vi "PathSup2ScanXML.vi"(3 "Thickness":dbl, 4 "Path":path, 5 "PathSupremes":T7[](array[typedef])) -> (2 "SCAN":T4)   [LabVIEW 2014]
uses:
  TypeDefs/PathSupreme.ctl
  Sub/VelocityProfile.ctl
  Sub/PathCut.ctl
  Sub/Segment.ctl
  TypeDefs/SCAN_XML.ctl
  Sub/Trajectory.ctl
  Sub/Path.ctl
  Sub/Point.ctl
  <vilib>/Utility/xml.llb/Write to XML File(string).vi
panel:
  out "xml string":string
  out "Path Supreames 2  String":string
  out "Trajectories Out":cluster{"TravelerID":u32, "SyncDelay":u32, T1[]}
  in  "SyncDelay":u32
  in  "TravelerID":u32
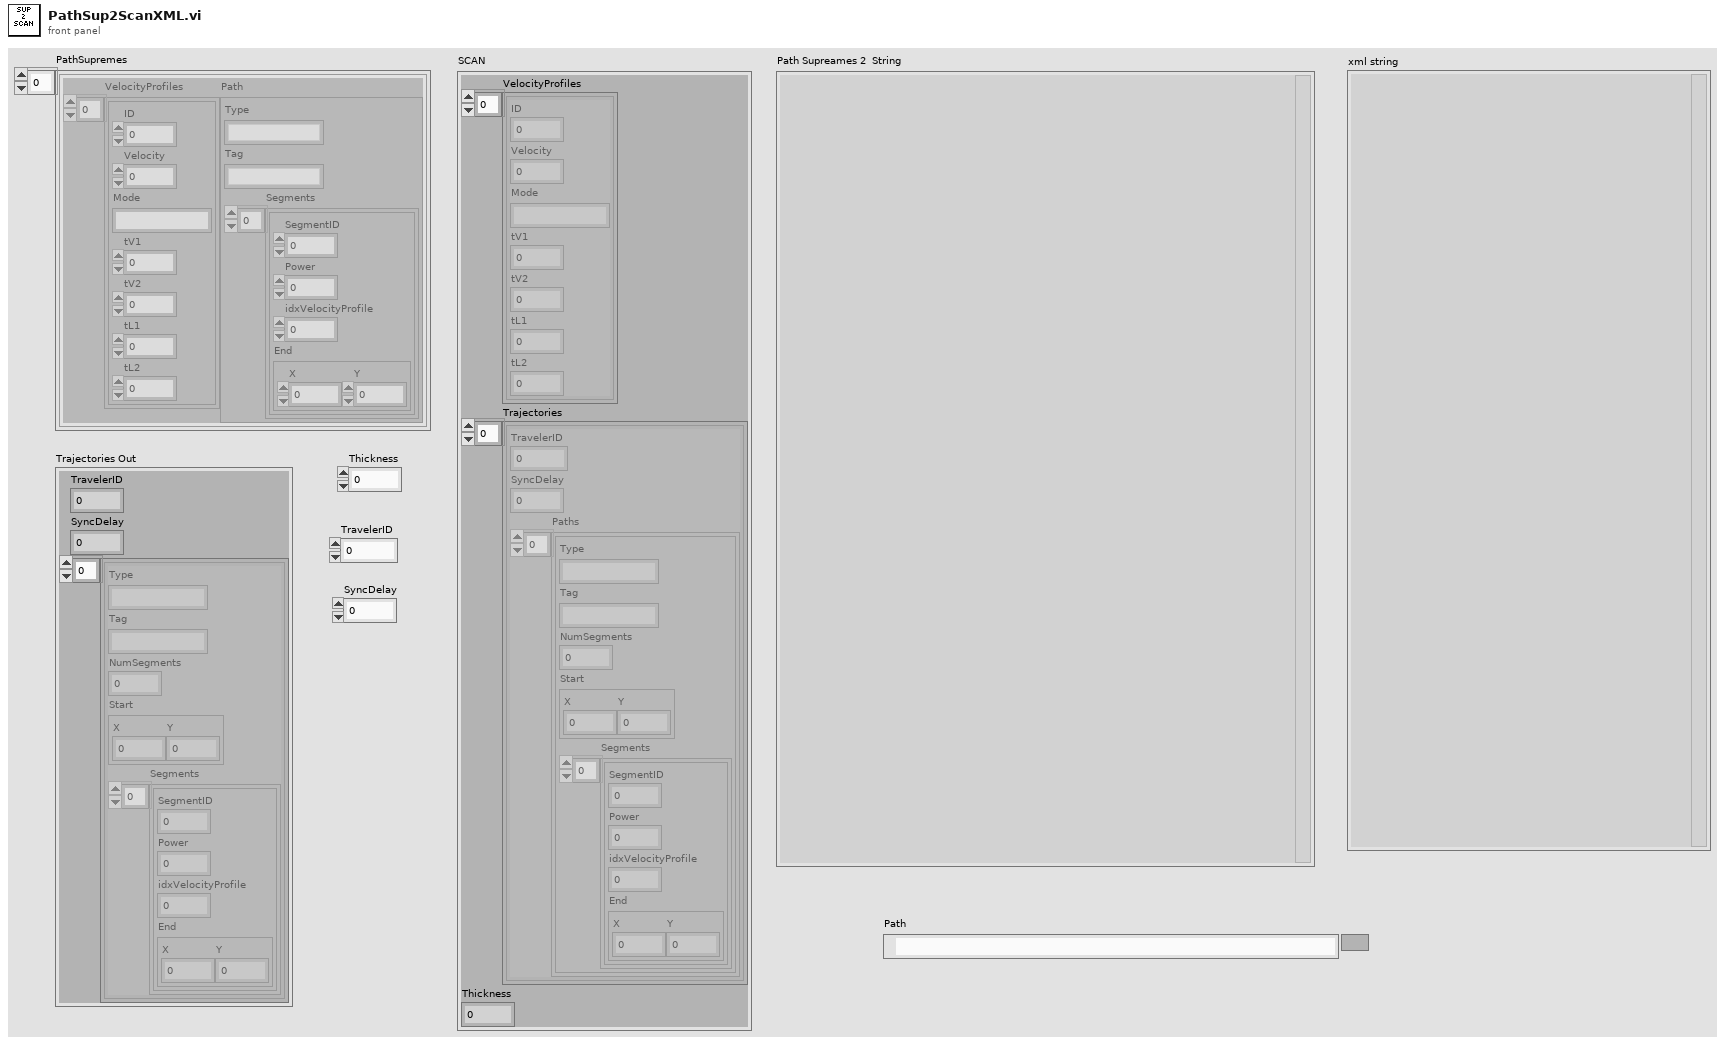
[diagram p1: front panel]
types:
  T1 = typedef "Path.ctl" = cluster{"Type":string, "Tag":string, "NumSegments":u64, "Start":T2, "Segments":T3[]}
  T2 = typedef "Point.ctl" = cluster{"X":dbl, "Y":dbl}
  T3 = typedef "Segment.ctl" = cluster{"SegmentID":u16, "Power":sgl, "idxVelocityProfile":u16, "End":cluster{"X":sgl, "Y":sgl}}
  T4 = typedef "SCAN_XML.ctl" = cluster{"VelocityProfiles":T5[], "Trajectories":T6[], "Thickness":dbl}
  T5 = typedef "VelocityProfile.ctl" = cluster{"ID":u32, "Velocity":dbl, "Mode":string, "tV1":u32, "tV2":u32, "tL1":u32, "tL2":u32}
  T6 = typedef "Trajectory.ctl" = cluster{"TravelerID":u32, "SyncDelay":u32, "Paths":T1[]}
  T7 = typedef "PathSupreme.ctl" = cluster{"VelocityProfiles":T5[], "Path":T8}
  T8 = typedef "PathCut.ctl" = cluster{"Type":string, "Tag":string, "Segments":T3[]}
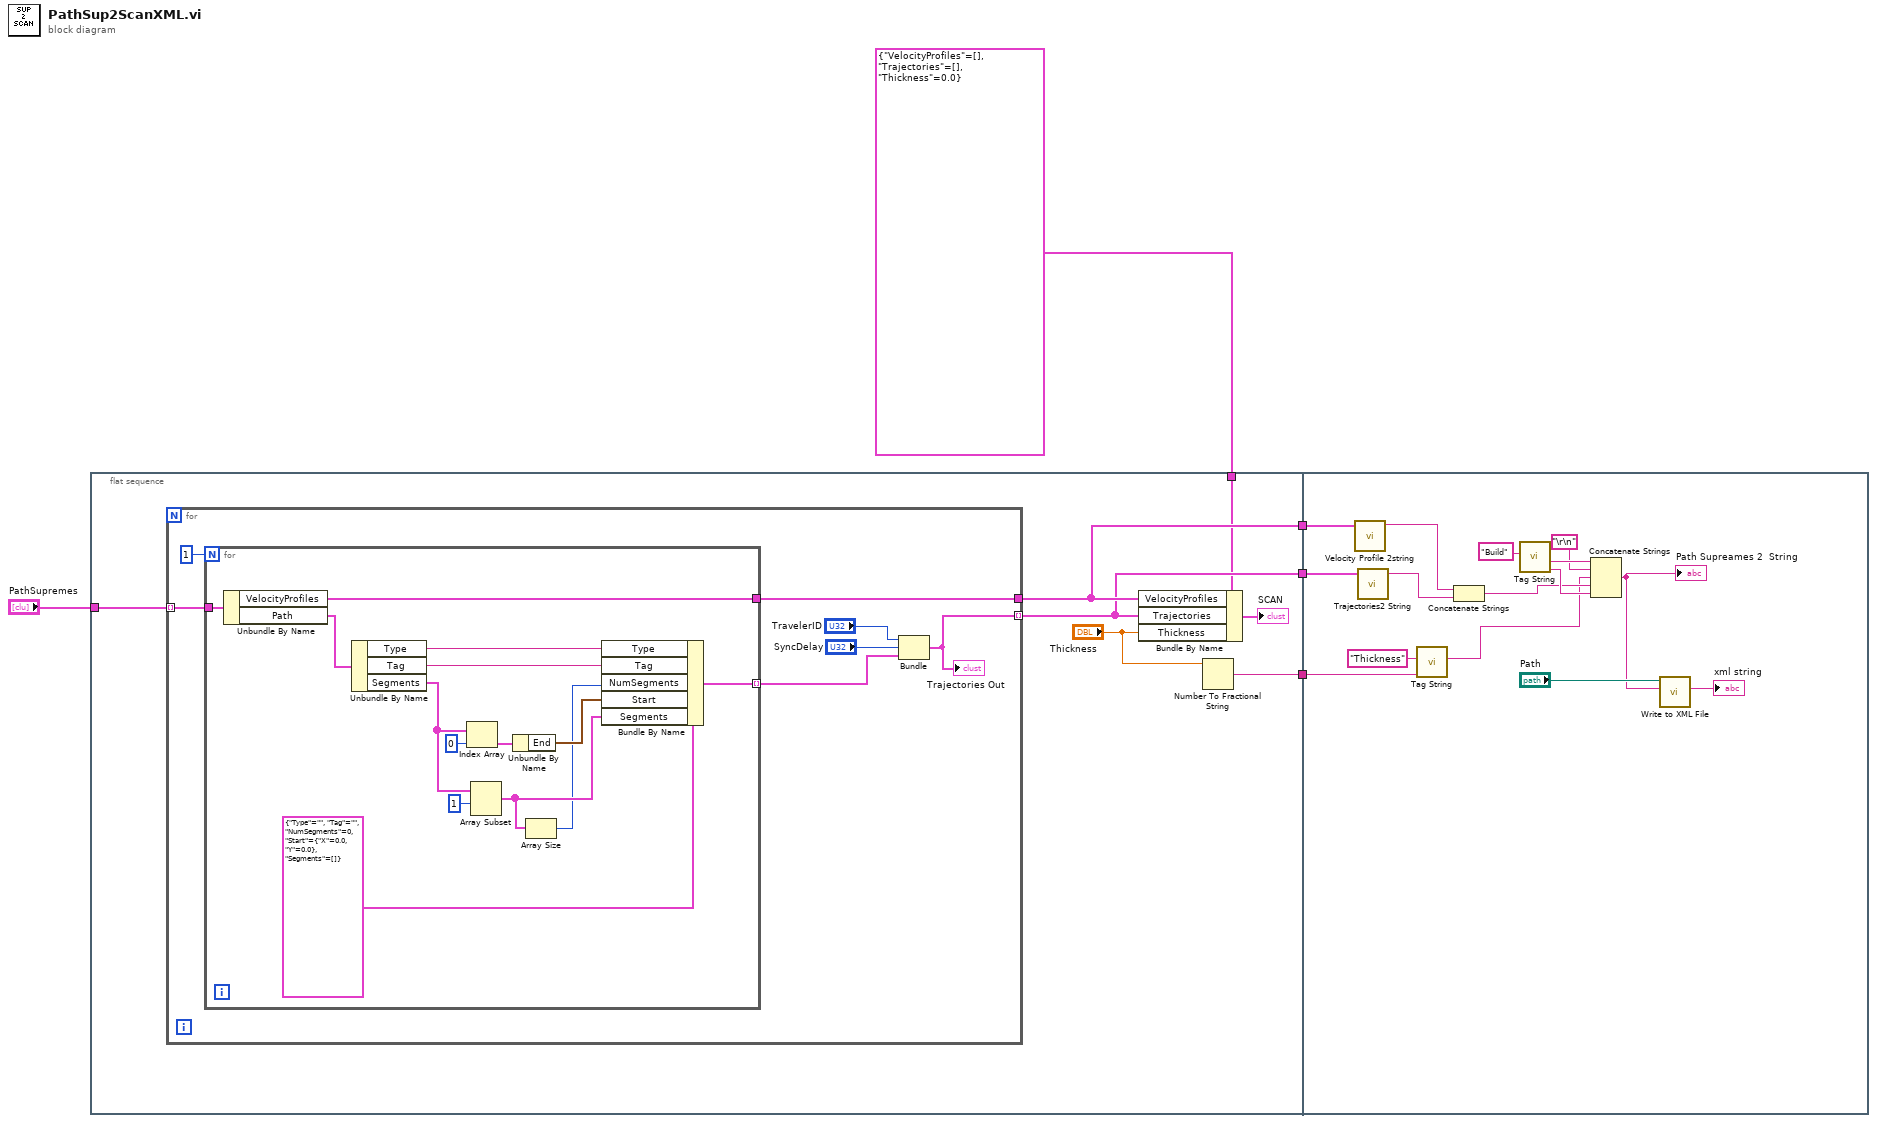
[diagram p0: block diagram]
diagram:
  n1 = flat-sequence {
    tunnel: "PathSupremes" -> [w12]
    tunnel: [w11] -> w4
    tunnel: [w10] -> w3
    tunnel: T4 {"VelocityProfiles"=[], "Trajectories"=[], "Thickness"=0.0} ("SCAN") -> [w9]
    tunnel: [w6] -> w1
    tunnel: w4 -> [w47]
    tunnel: w3 -> [w46]
    tunnel: w1 -> [w36]
    frame #0 {
      n2 = for {
        tunnel: w12 -> [w19] mode=indexing
        tunnel: [w18] -> w11
        tunnel: [w17] -> w10 mode=indexing
        n3 = for {
          N: 1 -> [_]
          tunnel: w19 -> [w33]
          tunnel: [w32] -> w18
          tunnel: [w22] -> w15 mode=indexing
          n4 = Unbundle By Name(w33) -> ("VelocityProfiles"=w32:T5[], "Path"=w30:T8)
          n5 = Unbundle By Name(w30) -> ("Type"=w29:string, "Tag"=w28:string, "Segments"=w25:T3[])
          n6 = Index Array(array=w25, index=0) -> (element=w26:T3)
          n7 = Array Subset(array=w25, index=1) -> (w21:T3[])  [unwired: 1 in]
          n8 = Unbundle By Name(w26) -> ("End"=w23:cluster{"X":sgl, "Y":sgl})
          n9 = Array Size(array=w21) -> (size(s)=w20:i32)
          n10 = Bundle By Name(cluster=T1 {"Type"="", "Tag"="", "NumSegments"=0, "Start"={"X"=0.0, "Y"=0.0}, "Segments"=[]} ("Path"), "Type"=w29, "Tag"=w28, "NumSegments"=w20, "Start"=w23, "Segments"=w21) -> (w22:T1)
        }
        n11 = Bundle("TravelerID"="TravelerID", "SyncDelay"="SyncDelay", w15) -> (w17:cluster{"TravelerID":u32, "SyncDelay":u32, T1[]})  [unwired: 1 in]
        "Trajectories Out" <- w17
      }
      n12 = Bundle By Name(cluster=w9, "VelocityProfiles"=w11, "Trajectories"=w10, "Thickness"="Thickness") -> (→"SCAN":T4)
      n13 = Number To Fractional String(number="Thickness") -> (F-format string=w6:string)  [unwired: 3 in]
    }
    frame #1 {
      n14 = call "Velocity Profile 2string.vi"("VelocityProfiles"=w47) -> ("VPL"=w44:string)  [unwired: 4 in]
      n15 = call "Trajectories2 String.vi"("Trajectories"=w46) -> ("VPL"=w45:string)  [unwired: 4 in]
      n16 = call "Tag String.vi"("String In"=w36, "String name"="Thickness") -> ("Start Tagged String Out"=w34:string)  [unwired: 3 in, 2 out]
      n17 = Concatenate Strings(w44, w45) -> (w39:string)
      n18 = call "Tag String.vi"("String name"="Build") -> ("Stop"=w40:string, "Start"=w41:string)  [unwired: 4 in, 1 out]
      n19 = Concatenate Strings(w41, "\r\n", w34, w39, w40) -> (w38:string)
      "Path Supreames 2  String" <- w38
      n20 = call-poly <vilib>:"Write to XML File.vi"("XML Input"=w38, "XML File Path"="Path") -> ("XML String"=→"xml string":string)  [unwired: 7 in, 2 out]
    }
  }
